vi "Insert Info Data.vi"(7 "info data to insert":string, 8 "sections":string[](array[string]), 11 "info data":string) -> (0 "sections out":string[](array[string]), 3 "info data out":string)   [LabVIEW 2013, in "infolib.lvlib"]
doc: "Inserts info data string into existing info data string at desired section."
uses:
  infolib.lvlib
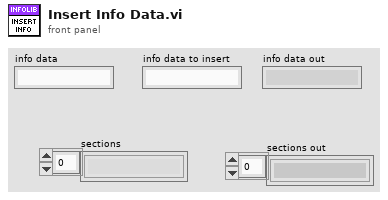
[diagram p1: front panel]
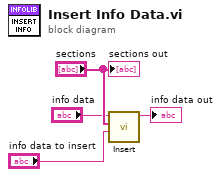
[diagram p0: block diagram]
diagram:
  n1 = call "Insert.vi"("insert"="info data to insert", "sections"="sections", "info data"="info data") -> ("info data out"=→"info data out":string)  [unwired: 8 in]
  "sections out" <- "sections"
